vi "ProcessFileFlow_Parse.vi"   [LabVIEW 2017, in "FileFlow.lvlib"]
doc: "Converts the in-memory TDMS file and properties from the previous process in the Fileflow Script from variant data to its original cluster format."
uses:
  <vilib>/addons/InsightCM/Devices/Shared/Common/FileFlow/FileFlow.lvlib
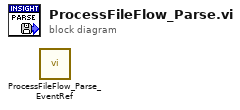
[diagram p0: block diagram]
diagram:
  n1 = call <vilib>:"ProcessFileFlow_Parse_EventRef.vi"() -> ()  [unwired: 10 in, 2 out]
